vi "MAINP Update BaudRate.vi"(7 "Controls":refnum<vi>[](array[refnum]), 8 "error in (no error)":errorcluster, 11 "Device Item Ref in":T1 format="%.0x") -> (0 "error out":errorcluster, 3 "Device Item Ref out":T1 format="%.0x")   [LabVIEW 2018, in "CAN Gateway System Explorer.lvlib"]
uses:
  CAN Gateway System Explorer.lvlib
  <vilib>/NI Veristand/Custom Device API/Custom Device Item Ref.ctl
  Types/BR Cluster.ctl
  Shared/Constants.vi
  <vilib>/NI Veristand/Custom Device API/Get Item Property (Variant).vi
  <vilib>/NI Veristand/Custom Device API/Custom Device API.lvlib
  Shared/CAN Gateway Shared.lvlib
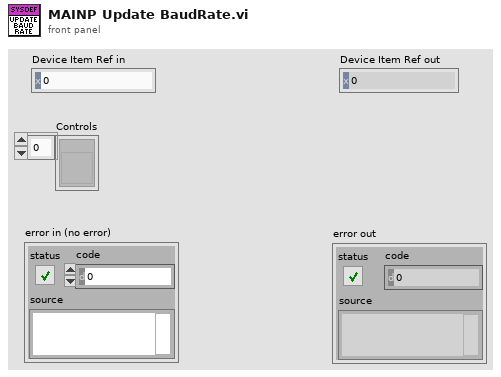
[diagram p1: front panel]
types:
  T1 = typedef "Custom Device API.lvlib/Custom Device Item Ref.ctl" = u64
  T2 = typedef "CAN Gateway System Explorer.lvlib/BR Cluster.ctl" = cluster{"BR Network-Port":u16, "BR Port Network":u16}
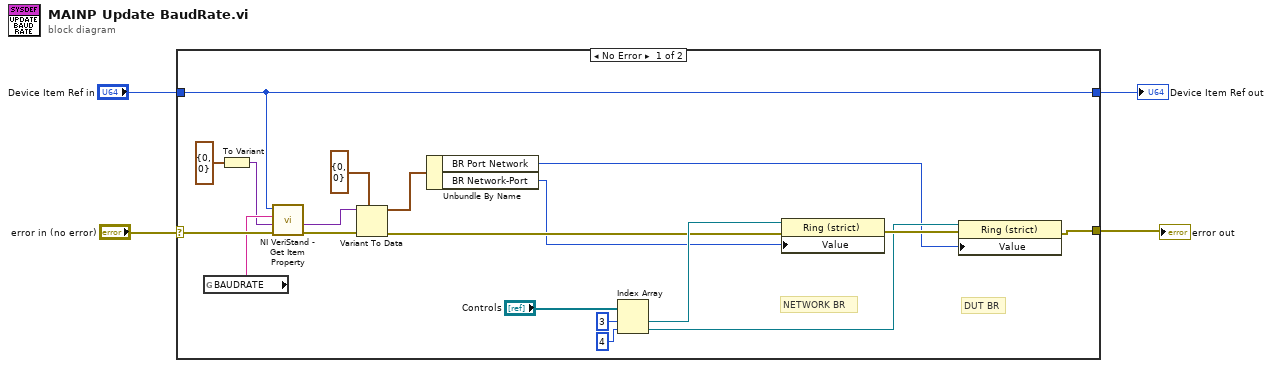
[diagram p0: block diagram]
diagram:
  n1 = case shown="No Error" "error in (no error)" {
    selector: "error in (no error)" -> [w23 w25]
    tunnel: "Device Item Ref in" -> [w21 w24]
    tunnel: [w21 w24] -> w2
    tunnel: [w18 w25] -> w1
    frame No Error {
      # "DUT BR"
      # "NETWORK BR"
      n2 = global read "Constants.vi" "BAUDRATE"() -> (w22:string)
      n3 = To Variant(anything=T2 {"BR Network-Port"=0, "BR Port Network"=0} ("BD Cluster")) -> (Variant=w5:variant)
      n4 = call-poly <vilib>:"NI VeriStand - Get Item Property.vi"("error in (no error)"=w23, "Default Value"=w5, "Property Name"=w22, "Item Ref in"=w21) -> ("error out"=w15:errorcluster, "Value"=w14:variant)  [unwired: 4 in, 2 out]
      n5 = Variant To Data(error in=w15, type=T2 {"BR Network-Port"=0, "BR Port Network"=0} ("BD Cluster"), Variant=w14) -> (data=w12:T2, error out=w11:errorcluster)
      n6 = Unbundle By Name(w12) -> ("BR Port Network"=w9:u16, "BR Network-Port"=w10:u16)
      n7 = Index Array(array="Controls", index #1=3 ("index"), index #2=4 ("index")) -> (element #1=w16:refnum<vi>, element #2=w17:refnum<vi>)
      n8 = property class="Ring (strict)"(reference=w16, error in=w11, "Value"=w10) -> (error out=w19:errorcluster)  [unwired: 1 out]
      n9 = property class="Ring (strict)"(reference=w17, error in=w19, "Value"=w9) -> (error out=w18:errorcluster)  [unwired: 1 out]
    }
    frame Error {
    }
  }
  "error out" <- w1
  "Device Item Ref out" <- w2
